vi "PH_Beamline_Chief.Event Call Set Settings.vi"(0 "VI in":refnum<vi>, 1 "Instance":string, 2 "Settings":T1, 5 "error in (no error)":errorcluster) -> (14 "VI out":refnum<vi>, 19 "error out":errorcluster)   [LabVIEW 2014, in "PH_Beamline_Chief.lvlib"]
uses:
  PH_Beamline_Chief.lvlib
  PH_Beamline_Chief.Settings.ctl
  CSCore/CSSystem/CoreLib/CoreLib.short 2 byte array.vi
  CSCore/CSSystem/CoreLib/CoreLib.lvlib
  CSCore/BaseProcess/BaseProcess.lvlib
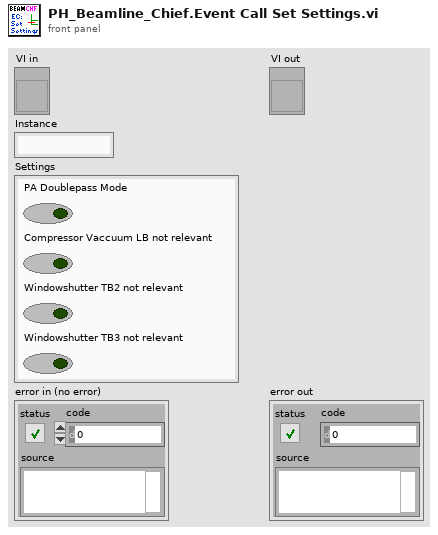
[diagram p1: front panel]
types:
  T1 = typedef "PH_Beamline_Chief.lvlib/PH_Beamline_Chief.Settings.ctl" = cluster{"PA Doublepass Mode":bool, "Compressor Vaccuum LB not relevant":bool, "Windowshutter TB2 not relevant":bool, "Windowshutter TB3 not relevant":bool}
  T2 = typedef "CoreDefs.rawDataType.ctl" = i8[]
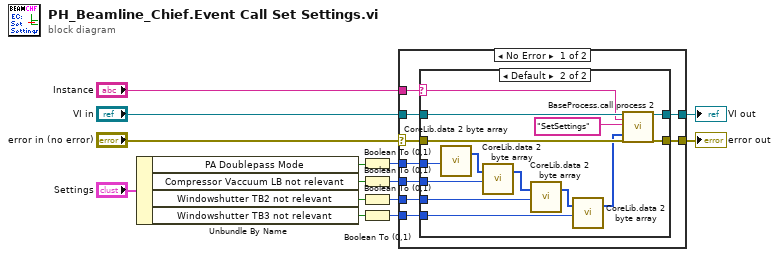
[diagram p0: block diagram]
diagram:
  n1 = Unbundle By Name("Settings") -> ("PA Doublepass Mode"=w8:bool, "Compressor Vaccuum LB not relevant"=w7:bool, "Windowshutter TB2 not relevant"=w6:bool, "Windowshutter TB3 not relevant"=w5:bool)
  n2 = Boolean To (0,1)(Boolean=w8) -> (0, 1=w4:i16)
  n3 = Boolean To (0,1)(Boolean=w7) -> (0, 1=w3:i16)
  n4 = Boolean To (0,1)(Boolean=w6) -> (0, 1=w2:i16)
  n5 = Boolean To (0,1)(Boolean=w5) -> (0, 1=w1:i16)
  n6 = case shown="No Error" "error in (no error)" {
    selector: "error in (no error)" -> [w19 w40]
    tunnel: [w23 w41] -> w13
    tunnel: [w22 w40] -> w12
    tunnel: "VI in" -> [w21 w41]
    tunnel: "Instance" -> [w20 _]
    tunnel: w4 -> [w18 _]
    tunnel: w3 -> [w17 _]
    tunnel: w2 -> [w16 _]
    tunnel: w1 -> [w15 _]
    frame No Error {
      n7 = case shown="Default" w20 {
        selector: w20 -> [_ w34]
        tunnel: [w25 w39] -> w23
        tunnel: [w24 w38] -> w22
        tunnel: w21 -> [w25 w37]
        tunnel: w19 -> [w24 w36]
        tunnel: w18 -> [_ w32]
        tunnel: w17 -> [_ w31]
        tunnel: w16 -> [_ w29]
        tunnel: w15 -> [_ w28]
        frame "N/A" {
        }
        frame Default {
          n8 = call-poly "CoreLib.data 2 byte array.vi"("i16"=w32) -> ("byteArray out"=w33:T2)  [unwired: 18 in]
          n9 = call-poly "CoreLib.data 2 byte array.vi"("byteArray"=w33, "i16"=w31) -> ("byteArray out"=w27:T2)  [unwired: 17 in]
          n10 = call-poly "CoreLib.data 2 byte array.vi"("byteArray"=w27, "i16"=w29) -> ("byteArray out"=w30:T2)  [unwired: 17 in]
          n11 = call-poly "CoreLib.data 2 byte array.vi"("byteArray"=w30, "i16"=w28) -> ("byteArray out"=w26:T2)  [unwired: 17 in]
          n12 = call "BaseProcess.call process 2.vi"("i ref in"=w37, "Object"=w34, "Selector"="SetSettings", "Data"=w26, "error in (no error)"=w36) -> ("i ref out"=w39:refnum<vi>, "error out"=w38:errorcluster)  [unwired: 13 in]
        }
      }
    }
    frame Error {
    }
  }
  "error out" <- w12
  "VI out" <- w13
